vi "Read RAW-Streamed File.vi"(8 "error in (no error)":errorcluster, 11 "Channel File 3":cluster{"File Path":path, "Simulate Data":bool}) -> (0 "error out":errorcluster, 3 "Array":waveform(cdb)[](array[waveform]))   [LabVIEW 2016]
panel:
  in  "Sampling Rate in MHz":dbl=100000000.0
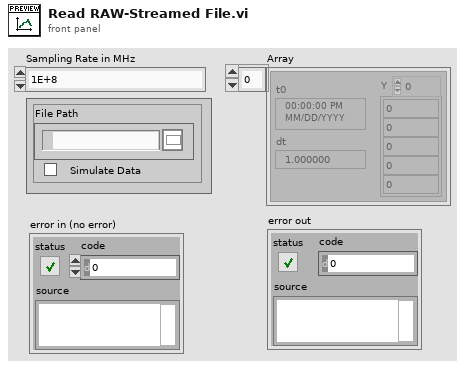
[diagram p1: front panel]
types:
  T1 = enum16{"open", "open or create", "create or replace", "create", "open (read-only)"}
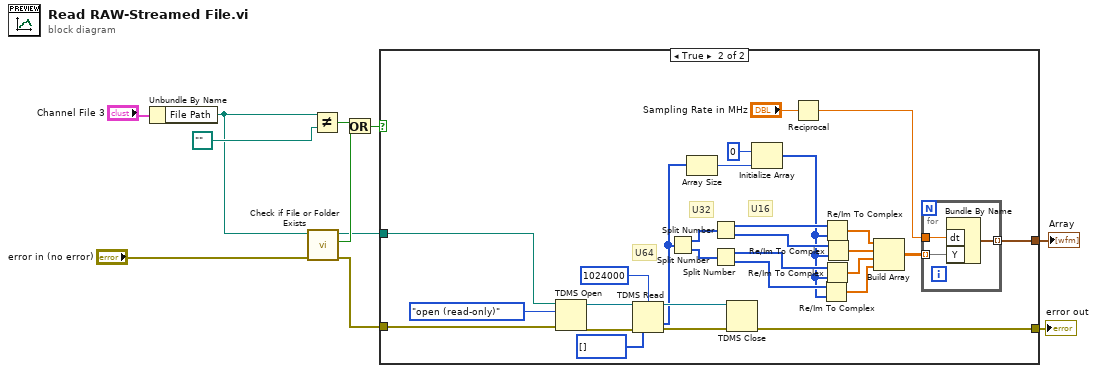
[diagram p0: block diagram]
diagram:
  n1 = Unbundle By Name("Channel File 3") -> ("File Path"=w2:path)
  n2 = call <vilib>:"Check if File or Folder Exists.vi"("error in (no error)"="error in (no error)", "path"=w2) -> ("error out"=w5:errorcluster, "file or folder exists?"=w6:bool, "dup path"=w4:path)  [unwired: 7 in]
  n3 = Not Equal?(x=w2, y=path "") -> (x != y?=w8:bool)
  n4 = Or(x=w8, y=w6) -> (x .or. y?=w7:bool)
  n5 = case shown="True" w7 {
    tunnel: w5 -> [w12 w40]
    tunnel: w4 -> [_ w39]
    tunnel: [w12 w22] -> w10
    tunnel: [_ w14] -> w1
    frame False {
    }
    frame True {
      # "U16"
      # "U32"
      # "U64"
      n6 = TDMS Open(8:w40, 10:T1."open (read-only)" ("operation (0:open)"), 11:w39) -> (0:w36:errorcluster, 3:w37:refnum<k34>)  [unwired: 4 in]
      n7 = TDMS Read(0:w37, 2:i64 1024000 ("count (-1: all)"), 11:w36, 12:u64[] []) -> (4:w35:refnum<k34>, 10:w30:u64[], 15:w34:errorcluster)  [unwired: 4 in, 3 out]
      n8 = Split Number(x=w30) -> (hi(x)=w32:u32[], lo(x)=w31:u32[])
      n9 = Array Size(array=w30) -> (size(s)=w29:i32)
      n10 = Split Number(x=w32) -> (hi(x)=w27:u16[], lo(x)=w26:u16[])
      n11 = Split Number(x=w31) -> (hi(x)=w25:u16[], lo(x)=w24:u16[])
      n12 = TDMS Close(8:w34, 11:w35) -> (0:w22:errorcluster)  [unwired: 1 out]
      n13 = Initialize Array(u16 0, w29) -> (w23:u16[])
      n14 = Reciprocal(x="Sampling Rate in MHz") -> (1/x=w15:dbl)
      n15 = Re/Im To Complex(1:w23, 2:w24) -> (0:w17:cdb[])
      n16 = Re/Im To Complex(1:w23, 2:w27) -> (0:w20:cdb[])
      n17 = Re/Im To Complex(1:w23, 2:w25) -> (0:w18:cdb[])
      n18 = Re/Im To Complex(1:w23, 2:w26) -> (0:w19:cdb[])
      n19 = Build Array(w20, w19, w18, w17) -> (w16:cdb[][])
      n20 = for {
        tunnel: w16 -> [w43] mode=indexing
        tunnel: w15 -> [w42]
        tunnel: [w41] -> w14 mode=indexing
        n21 = Bundle By Name("dt"=w42, "Y"=w43) -> (w41:waveform(cdb))  [unwired: 1 in]
      }
    }
  }
  "error out" <- w10
  "Array" <- w1
